vi "TurnSpeedAdjust.vi"(9 "Turn":dbl format="%#_13g", 10 "Y":dbl format="%#_13g", 11 "X":dbl format="%#_13g") -> (3 "TurnAdjusted":dbl)   [LabVIEW 2018]
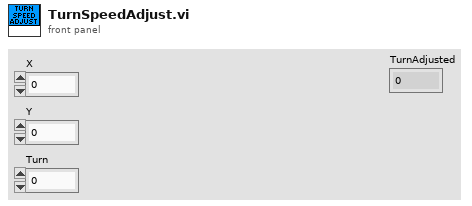
[diagram p1: front panel]
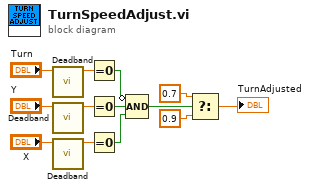
[diagram p0: block diagram]
diagram:
  n1 = call "Deadband.vi"("Input"="Turn") -> ("Output"=w10:dbl)  [unwired: 6 in]
  n2 = call "Deadband.vi"("Input"="Y") -> ("Output"=w9:dbl)  [unwired: 6 in]
  n3 = call "Deadband.vi"("Input"="X") -> ("Output"=w8:dbl)  [unwired: 6 in]
  n4 = Equal To 0?(x=w10) -> (x = 0?=w7:bool)
  n5 = Equal To 0?(x=w9) -> (x = 0?=w6:bool)
  n6 = Equal To 0?(x=w8) -> (x = 0?=w5:bool)
  n7 = Compound Arithmetic op=AND(invert w7, w6, w5) -> (w4:bool)
  n8 = Select(t=0.7, s=w4, f=0.9) -> (s? t:f=→"TurnAdjusted":dbl)
